vi "Register Main Panel.vi"(8 "error in (no error)":errorcluster, 10 "TableName":string, 11 "Login.lvclass":refnum<class "Login.lvclass">) -> (0 "error out":errorcluster, 3 "Login out":refnum<class "Login.lvclass">)   [LabVIEW 2015, in "Login.lvclass"]
uses:
  Login.lvclass
panel:
  in  "真实姓名":string
  in  "Register":bool
  in  "学号":string
  in  "再输入一次密码":string
  in  "密码":string
  in  "用户名":string
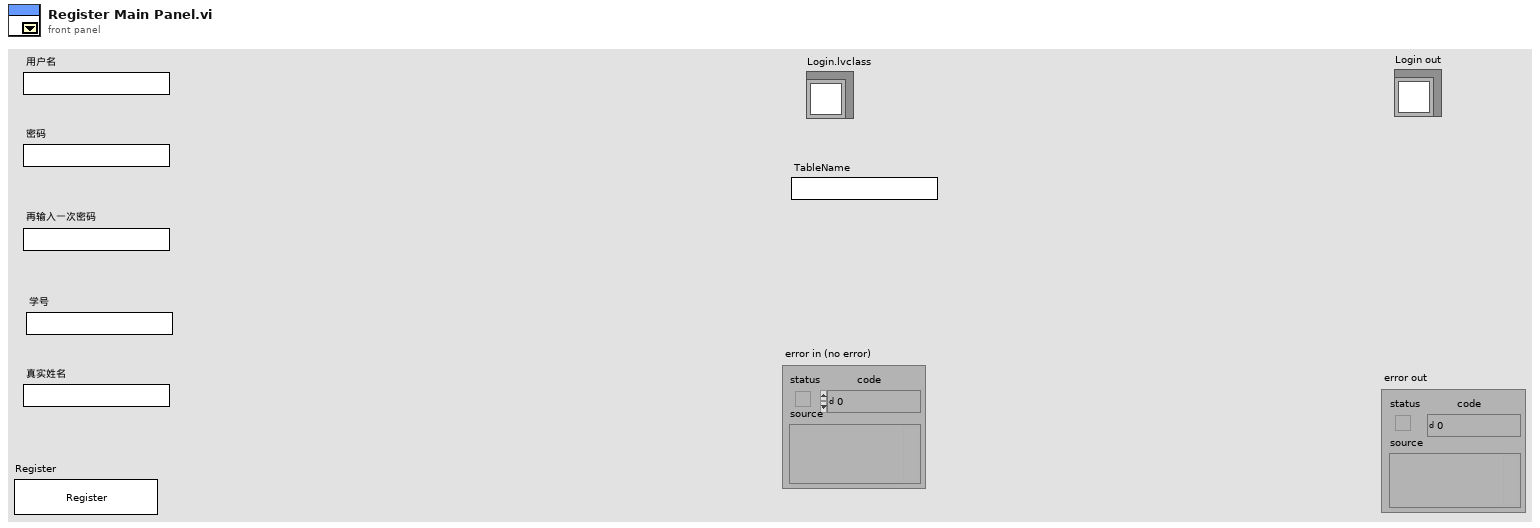
[diagram p1: front panel]
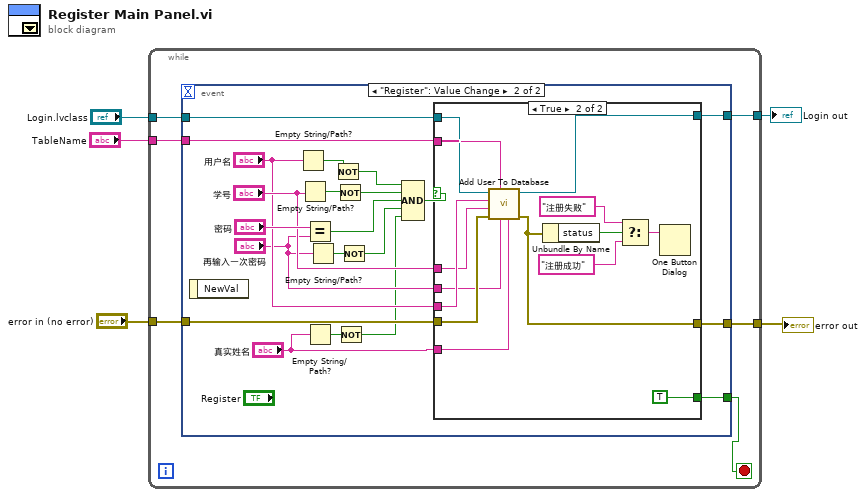
[diagram p0: block diagram]
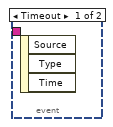
[diagram p2: hidden frame]
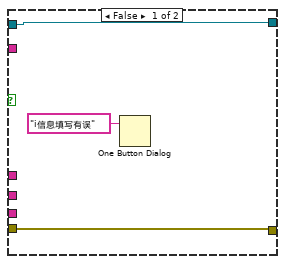
[diagram p3: hidden frame]
diagram:
  n1 = while {
    tunnel: "Login.lvclass" -> [w11]
    tunnel: "error in (no error)" -> [w10]
    tunnel: "TableName" -> [w9]
    tunnel: [w8] -> w1
    tunnel: [w7] -> w2
    stop <- w6 stop-if-true
    n2 = event shown="[1] \"Register\": Value Change" {
      selector: _ -> [_ _]
      dyn-events: _ -> [_ _]
      timeout: _ -> [_ _]
      tunnel: w11 -> [_ w25]
      tunnel: w10 -> [_ w24]
      tunnel: w9 -> [_ w21]
      tunnel: [_ w20] -> w8
      tunnel: [_ w19] -> w7
      tunnel: [_ w18] -> w6
      event Timeout {
        n3 = event-data() -> ()  [unwired: 1 in, 3 out]
      }
      event "Register": Value Change {
        n4 = event-data() -> ()  [unwired: 1 in, 1 out]
        n5 = Empty String/Path?(string/path="用户名") -> (empty?=w32:bool)
        n6 = Empty String/Path?(string/path="学号") -> (empty?=w31:bool)
        n7 = Equal?(x="密码", y="再输入一次密码") -> (x = y?=w27:bool)
        n8 = Empty String/Path?(string/path="真实姓名") -> (empty?=w14:bool)
        n9 = Empty String/Path?(string/path="再输入一次密码") -> (empty?=w16:bool)
        n10 = Not(x=w32) -> (.not. x?=w29:bool)
        n11 = Not(x=w31) -> (.not. x?=w28:bool)
        n12 = Not(x=w14) -> (.not. x?=w13:bool)
        n13 = Not(x=w16) -> (.not. x?=w15:bool)
        n14 = Compound Arithmetic op=AND(w29, w28, w27, w15, w13) -> (w26:bool)
        n15 = case shown="True" w26 {
          tunnel: w25 -> [w34 w49]
          tunnel: w24 -> [w35 w46]
          tunnel: "学号" -> [_ w47]
          tunnel: "再输入一次密码" -> [_ w45]
          tunnel: "用户名" -> [_ w48]
          tunnel: w21 -> [_ w44]
          tunnel: [w34 w43] -> w19
          tunnel: [w35 w42] -> w20
          tunnel: [_ TRUE] -> w18
          tunnel: "真实姓名" -> [_ w36]
          frame False {
            n16 = One Button Dialog(message="i信息填写有误") -> ()  [unwired: 1 in, 1 out]
          }
          frame True {
            n17 = call "Add User To Database.vi"("Name(\"\")"=w36, "Pwd(\"\")"=w45, "Table(\"\")"=w44, "error in (no error)"=w46, "ID(\"\")"=w47, "UserName(\"\")"=w48, "Login in"=w49) -> ("error out"=w42:errorcluster, "Login out"=w43:refnum<class "Login.lvclass">)  [unwired: 3 in]
            n18 = Unbundle By Name(w42) -> ("status"=w41:bool)
            n19 = Select(t="注册失败", s=w41, f="注册成功") -> (s? t:f=w38:string)
            n20 = One Button Dialog(message=w38) -> ()  [unwired: 1 in, 1 out]
          }
        }
      }
    }
  }
  "error out" <- w1
  "Login out" <- w2
